vi "QTMDriver.vi"(0 "connection ID":refnum<k5>, 1 "Ring":T1, 5 "DataIn":dbl[](array[numeric]), 7 "QTMqueue":refnum<queue>, 9 "VI Refnum QTMTask":refnum<vi>, 11 "error in":errorcluster, 12 "timeout ms (25000)":i32=6000, 13 "DataOutIndex":i32=1) -> (3 "ArrayOut":dbl[](array[numeric]), 4 "connection ID out":refnum<k5>, 6 "DataOut":dbl[](array[numeric]), 8 "QTMqueue Out":refnum<queue>, 14 "VI Refnum QTMTask Out":refnum<vi>, 15 "error out":errorcluster)   [LabVIEW 2014, in "Oqus Custom Device.lvlib"]
uses:
  Oqus Custom Device.lvlib
  CustomIO.ctl
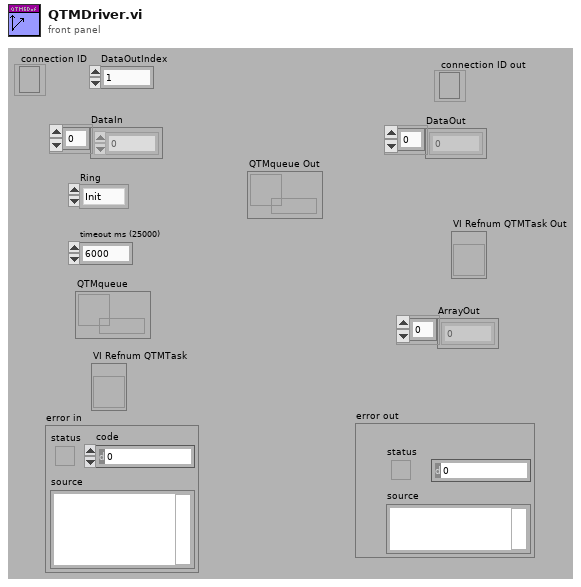
[diagram p1: front panel]
types:
  T1 = typedef "Oqus Custom Device.lvlib/CustomIO.ctl" = enum16{"Init", "Read", "Write", "Close", "N/O"}
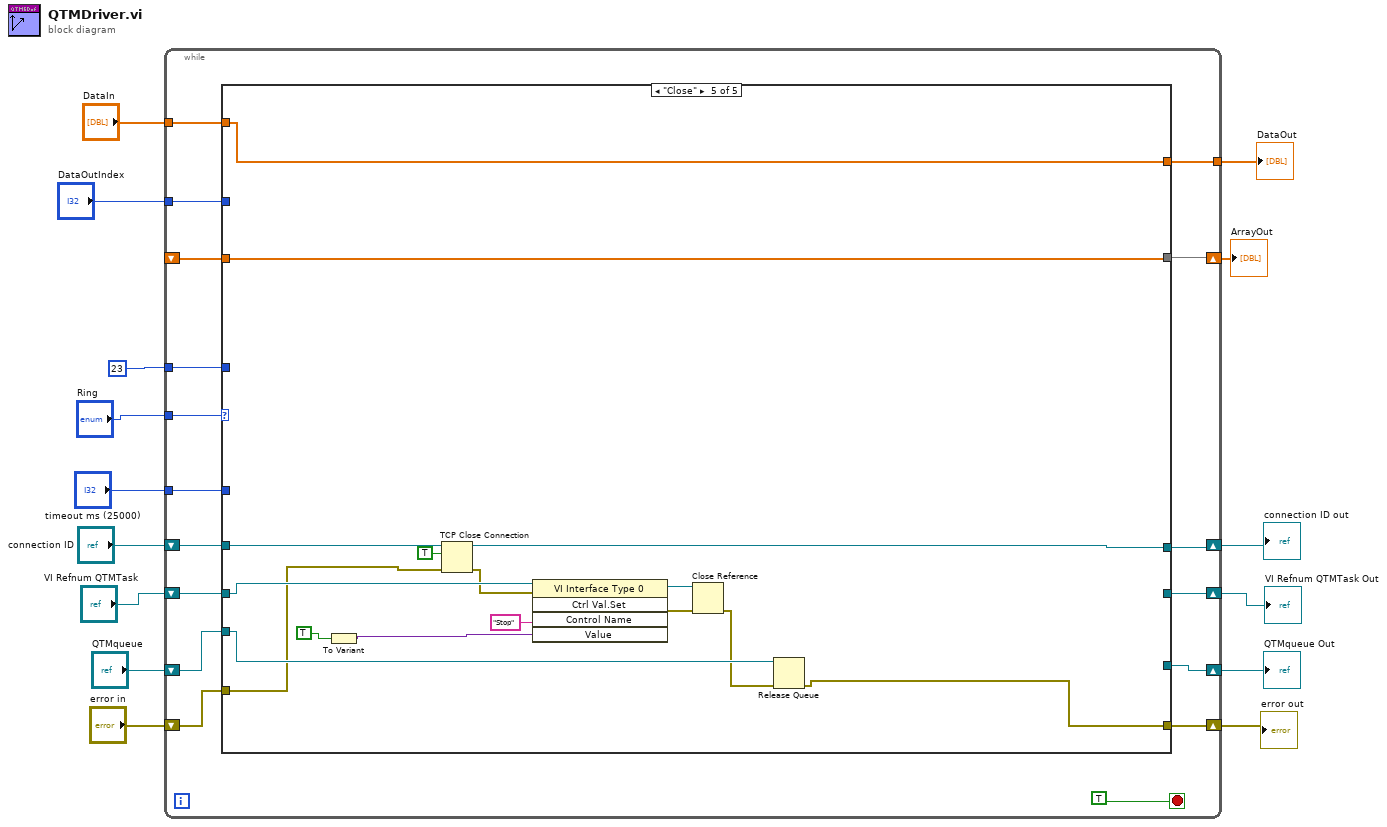
[diagram p0: block diagram]
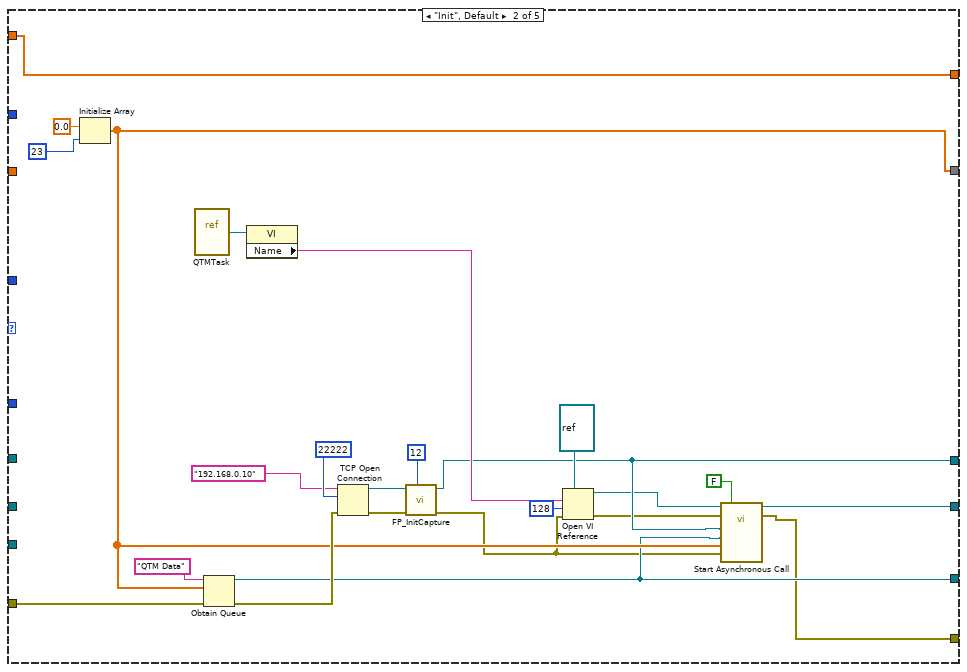
[diagram p3: hidden frame]
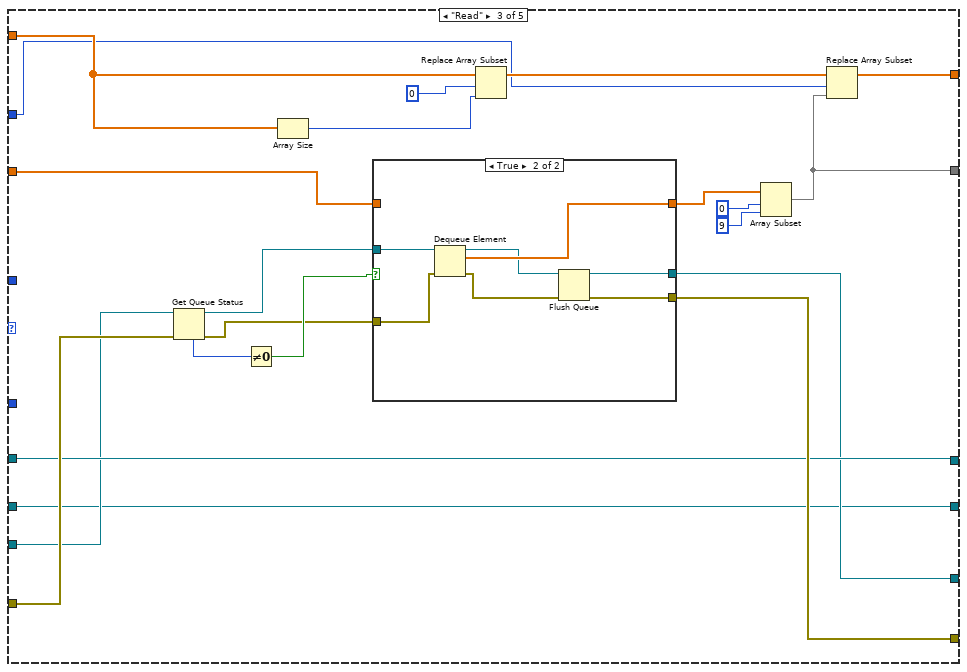
[diagram p4: hidden frame]
diagram:
  n1 = while {
    tunnel: "Ring" -> [w32]
    shift-right: [w31] -> w6
    shift-left: _ -> [w30]
    tunnel: 23 -> [w29]
    shift-right: [w27] -> w13
    shift-left: "error in" -> [w28]
    shift-right: [w25] -> w11
    shift-left: "connection ID" -> [w26]
    tunnel: "DataIn" -> [w24]
    tunnel: [w23] -> w9
    tunnel: "DataOutIndex" -> [w22]
    tunnel: "timeout ms (25000)" -> [w21]
    shift-right: [w20] -> w3
    shift-left: "QTMqueue" -> [w19]
    shift-right: [w18] -> w1
    shift-left: "VI Refnum QTMTask" -> [w17]
    stop <- TRUE stop-if-true
    n2 = case shown="\"Close\"" w32 {
      tunnel: [w38 w48 w63 w98 w113] -> w31
      tunnel: w30 -> [w38 _ w74 w98 w113]
      tunnel: w29 -> [_ _ _ _ _]
      tunnel: w28 -> [w37 w54 w77 w94 w100]
      tunnel: [w37 w39 w71 w94 w108] -> w27
      tunnel: w26 -> [w33 _ w70 w99 w115]
      tunnel: [w33 w46 w70 w99 w114] -> w25
      tunnel: w24 -> [w36 w58 w80 w97 w112]
      tunnel: [w36 w58 w79 w97 w112] -> w23
      tunnel: w22 -> [_ _ w78 _ _]
      tunnel: w21 -> [_ _ _ _ _]
      tunnel: [w35 w47 w68 w96 _] -> w20
      tunnel: w19 -> [w35 _ w69 w96 w110]
      tunnel: [w34 w45 w67 w95 _] -> w18
      tunnel: w17 -> [w34 _ w67 w95 w111]
      frame "N/O" {
      }
      frame "Init", Default {
        n3 = Initialize Array(0.0 ("element"), 23) -> (w48:dbl[])
        n4 = vi-ref "QTMTask.vi"() -> (w49:refnum<vi>)
        n5 = Obtain Queue(name (unnamed)="QTM Data", element data type=w48, error in (no error)=w54) -> (queue out=w47:refnum<queue>, error out=w53:errorcluster)  [unwired: 2 in, 1 out]
        n6 = property class="VI"(reference=w49) -> ("Name"=w51:string)  [unwired: 1 in, 2 out]
        n7 = TCP Open Connection(address="192.168.0.10", remote port or service name=u16 22222, error in (no error)=w53) -> (connection ID=w62:refnum<k5>, error out=w61:errorcluster)  [unwired: 2 in]
        n8 = call "FP_InitCapture.vi"("ComponentType"=u32 12, "error out 2"=w61, "connection ID"=w62) -> ("error out"=w41:errorcluster, "connection ID out"=w46:refnum<k5>)  [unwired: 5 in, 2 out]
        n9 = Open VI Reference(type specifier VI Refnum (for type only)=refnum<vi> refnum, vi path=w51, options=128, error in (no error)=w41) -> (vi reference=w43:refnum<vi>, error out=w42:errorcluster)  [unwired: 2 in]
        n10 = call-by-ref "Start Asynchronous Call"(reference=w43, error in=w42, "Stop"=FALSE, "error in"=w41, "ArrayIn"=w48, "QTMqueue"=w47, "connection ID"=w46) -> (reference out=w45:refnum<vi>, error out=w39:errorcluster)  [unwired: 4 in, 2 out]
      }
      frame "Read" {
        n11 = Get Queue Status(queue=w69, error in (no error)=w77) -> (queue out=w73:refnum<queue>, error out=w72:errorcluster, # elements in queue=w76:i32)  [unwired: 1 in, 5 out]
        n12 = Not Equal To 0?(x=w76) -> (x != 0?=w75:bool)
        n13 = Array Size(array=w80) -> (size(s)=w81:i32)
        n14 = case shown="True" w75 {
          tunnel: w74 -> [w86 _]
          tunnel: w73 -> [w84 w93]
          tunnel: [w86 w92] -> w64
          tunnel: w72 -> [w85 w89]
          tunnel: [w85 w88] -> w71
          tunnel: [w84 w87] -> w68
          frame False {
          }
          frame True {
            n15 = Dequeue Element(queue=w93, error in (no error)=w89) -> (queue out=w91:refnum<queue>, element=w92:dbl[], error out=w90:errorcluster)  [unwired: 1 in, 1 out]
            n16 = Flush Queue(queue=w91, error in (no error)=w90) -> (queue out=w87:refnum<queue>, error out=w88:errorcluster)  [unwired: 1 out]
          }
        }
        n17 = Replace Array Subset(array=w80, new element=w81, index=0) -> (w82:dbl[])
        n18 = Array Subset(array=w64, index=0, length=9) -> (w63:dbl[])
        n19 = Replace Array Subset(array=w82, new element=w63, index=w78) -> (w79:dbl[])
      }
      frame "Write" {
      }
      frame "Close" {
        n20 = To Variant(anything=TRUE) -> (Variant=w104:variant)
        n21 = TCP Close Connection(connection ID=w115, abort (F)=TRUE, error in (no error)=w100) -> (connection ID out=w114:refnum<k5>, error out=w102:errorcluster)
        n22 = invoke class="VI Interface Type 0" method="Ctrl Val.Set"(reference=w111, error in=w102, "Control Name"="Stop", "Value"=w104) -> (reference out=w107:refnum<vi>, error out=w101:errorcluster)  [unwired: 1 in, 3 out]
        n23 = Close Reference(reference=w107, error in (no error)=w101) -> (error out=w109:errorcluster)
        n24 = Release Queue(queue=w110, error in (no error)=w109) -> (error out=w108:errorcluster)  [unwired: 1 in, 2 out]
      }
    }
  }
  "error out" <- w13
  "connection ID out" <- w11
  "DataOut" <- w9
  "ArrayOut" <- w6
  "QTMqueue Out" <- w3
  "VI Refnum QTMTask Out" <- w1
